vi "Sound Devices Numbers.vi"() -> ()   [LabVIEW 2019]
panel:
  out "Input\nDevices":string[](array[string])
  out "Input\nCapabilities":T1(array[cluster])
  out "Output\nCapabilities":T1(array[cluster])
  out "Output\nDevices":string[](array[string])
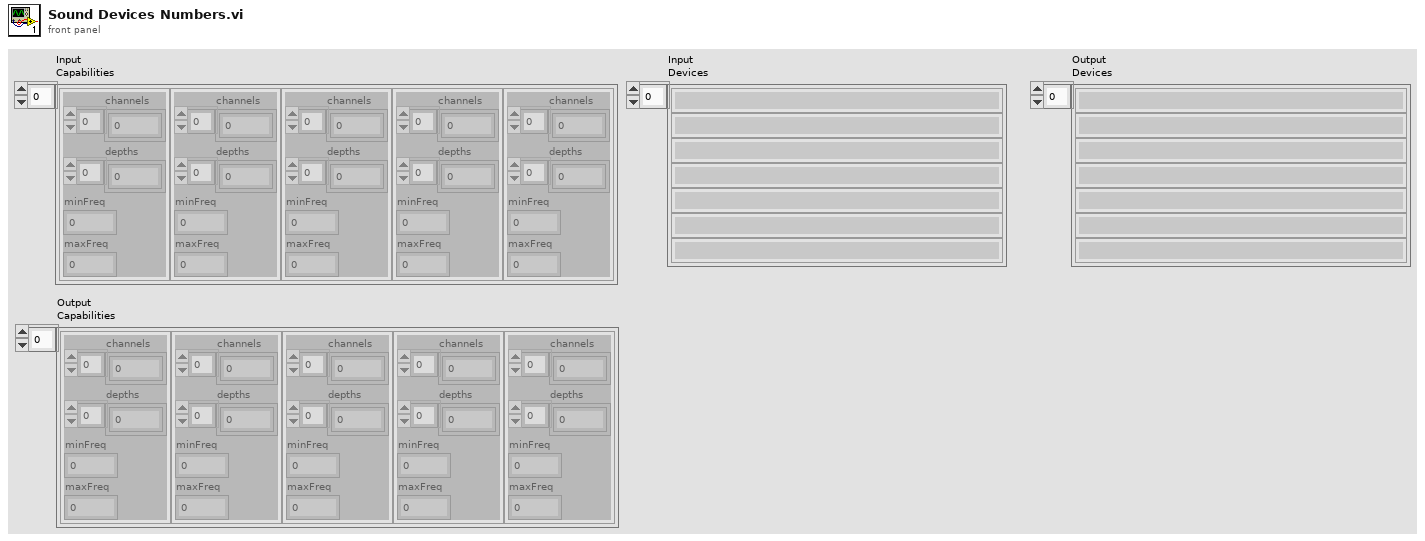
[diagram p1: front panel]
types:
  T1 = cluster{"channels":i32[], "depths":i32[], "minFreq":dbl, "maxFreq":dbl}[]
  T2 = cluster{"channels":i32[], "depths":i32[], "minFreq":dbl, "maxFreq":dbl}
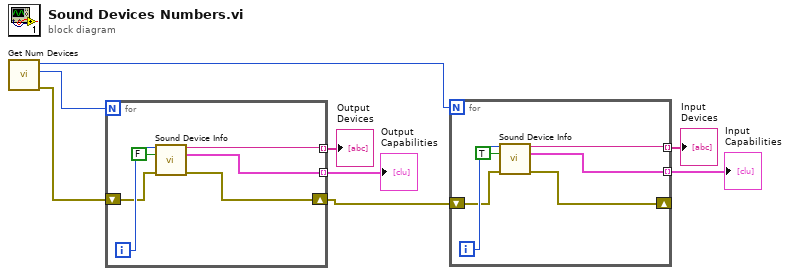
[diagram p0: block diagram]
diagram:
  n1 = call <vilib>:"Get Num Devices.vi"() -> ("error out"=w2:errorcluster, "Number of Output Devices"=w8:i32, "Number of Input Devices"=w3:i32)  [unwired: 9 in]
  n2 = for {
    N: w8 -> [_]
    tunnel: [w12] -> w7 mode=indexing
    tunnel: [w11] -> w6 mode=indexing
    shift-right: [w9] -> w1
    shift-left: w2 -> [w10]
    i -> [w14]
    n3 = call <vilib>:"Sound Device Info.vi"("device"=w14, "isInput?"=FALSE, "error in (no error)"=w10) -> ("Device Name"=w12:string, "Capabilities"=w11:T2, "error out"=w9:errorcluster)  [unwired: 10 in]
  }
  "Output\nDevices" <- w7
  "Output\nCapabilities" <- w6
  n4 = for {
    N: w3 -> [_]
    tunnel: [w18] -> w4 mode=indexing
    tunnel: [w17] -> w5 mode=indexing
    shift-right: [w15] -> _
    shift-left: w1 -> [w16]
    i -> [w20]
    n5 = call <vilib>:"Sound Device Info.vi"("device"=w20, "isInput?"=TRUE, "error in (no error)"=w16) -> ("Device Name"=w18:string, "Capabilities"=w17:T2, "error out"=w15:errorcluster)  [unwired: 10 in]
  }
  "Input\nDevices" <- w4
  "Input\nCapabilities" <- w5
